vi "goToHome.vi"(0 "Controller in":refnum<class "_Controller.lvclass">, 1 "axis (for multi-axis applications only)":T2, 2 "dir":T1, 3 "mode (for multi-axis applications only)":T3, 5 "error in (no error)":errorcluster) -> (14 "Controller out":refnum<class "_Controller.lvclass">, 17 "success?":bool, 18 "response":string, 19 "error out":errorcluster)   [LabVIEW 2013, in "classes.lvlib" / "_Controller.lvclass"]
doc: "Jog to the Home Limit position for a given axis. For single axis applications, axis need not be specified.\n\nProduced By:\n\n<B>Kod Integrations, LLC</B>\n4835 Marianne Drive\nMount Airy, MD 21771\nhttp://www.kodintegrations.com\nemail: info@kodintegrations.com\nphone: (240) 687-1288"
uses:
  _Controller.lvclass
  homing_mode.ctl
  axis.ctl
  linear_direction.ctl
  common.lvlib
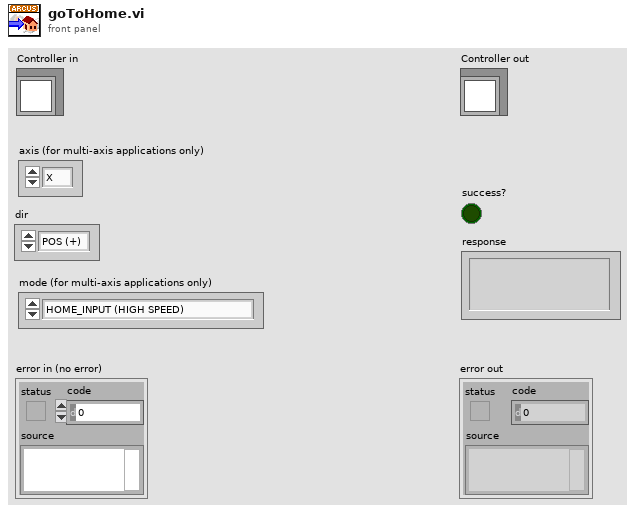
[diagram p1: front panel]
types:
  T1 = typedef "common.lvlib/linear_direction.ctl" = enum16{"POS (+)", "NEG (-)"}
  T2 = typedef "common.lvlib/axis.ctl" = enum16{"X", "Y", "Z", "U"}
  T3 = typedef "common.lvlib/homing_mode.ctl" = enum16{"HOME_INPUT (HIGH SPEED)", "LIMIT_INPUT", "HOME_INPUT_&_Z-INDEX", "Z-INDEX", "HOME_INPUT (HIGH_&_LOW_SPEED)"}
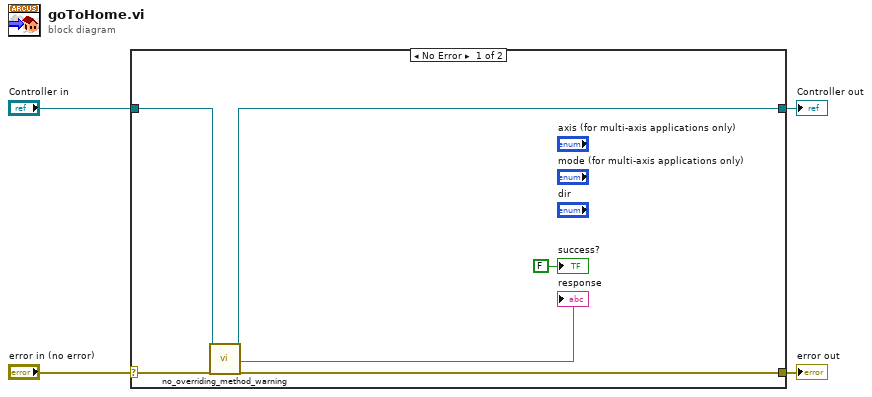
[diagram p0: block diagram]
diagram:
  n1 = case shown="No Error" "error in (no error)" {
    selector: "error in (no error)" -> [w9 w12]
    tunnel: [w8 w12] -> w3
    tunnel: [w6 w11] -> w1
    tunnel: "Controller in" -> [w7 w11]
    frame No Error {
      n2 = call "no_overriding_method_warning.vi"("Controller (in)"=w7, "error in (no error)"=w9) -> ("Controller (out)"=w6:refnum<class "_Controller.lvclass">, "msg"=→"response":string, "error out"=w8:errorcluster)  [unwired: 15 in]
      "success?" <- FALSE ("success?")
    }
    frame Error {
    }
  }
  "error out" <- w3
  "Controller out" <- w1
